vi "initalize 6221-2182-dc(SubVI).vi"(9 "字符串":string, 11 "簇":T13={"initialize"=enum."SR830", "6221"={"6221 Resource"="GPIB0::24::INSTR", "Delta status"=FALSE, "电流"=0.0}, "SR830+6221"={"source"=0, "阻抗"=0.0, "量程入 4"=0, "量程入 3"=0, "量程入 2"=0, "量程入 1"=0, "SR830 2"=FALSE, "SR830 3"=FALSE, "SR830 4"=FALSE, "SR830 1"=FALSE, "VISA 1"="", "VISA 2"="", "VISA 3"="", "VISA 4"="", "Reserve 1"=0, "Reserve 2"=-1, "Reserve 3"=-1, "Reserve 4"=-1, "量程"=enum."量程每次测量会判定"}, "2400"={"2400"=FALSE, "VISA"=""}, "ch"={"ch"=[], "current"=[], "change?"=[], "holding current\nwhen change ch?"=FALSE}, "Instrument"={"335 Resource"="GPIB0::24::INSTR", "Input (0:A)"=0, "Instrument Type"=enum."SVSM", "quantum design"=refnum, "Heater Output (1:1)"=1, "semaphore"=refnum, "TCP master instance"=refnum, "335 Status"=refnum, "M24C Resource"="GPIB0::24::INSTR", "4G supply"="GPIB0::24::INSTR", "Temp Status 24C"=refnum, "Temp"=refnum, "9T信号"=refnum, "limit"={"Field limit"=0.0, "Field rate limit"=0.0, "Temp limit"=0.0, "Temp low limit"=0.0, "Temp rate limit "=0.0}, "4g supply status"=refnum, "vi路径"=""}, "Aborting"=refnum, "数据文件"=refnum, "warning"=refnum, "2614B"={"2614B chA"=FALSE, "2614B chB"=FALSE, "VISA"=""}} {"Instrument"."Input (0:A)" items=["A", "B"]; "Instrument"."Heater Output (1:1)" items=["1"=1, "2"=2]; "SR830+6221"."Reserve 4" items=["Auto Reserve"=-1, "High Reserve"=0, "Normal"=1, "Low Noise"=2]; "SR830+6221"."Reserve 3" items=["Auto Reserve"=-1, "High Reserve"=0, "Normal"=1, "Low Noise"=2]; "SR830+6221"."Reserve 2" items=["Auto Reserve"=-1, "High Reserve"=0, "Normal"=1, "Low Noise"=2]; "SR830+6221"."Reserve 1" items=["量程每次测量会判定", "量程不变为设定值"]; "SR830+6221"."source" items=["SR830 1", "SR830 2", "SR830 3", "SR830 4"]}) -> (3 "输出簇":T13={"initialize"=enum."SR830", "6221"={"6221 Resource"="GPIB0::24::INSTR", "Delta status"=FALSE, "电流"=0.0}, "SR830+6221"={"source"=0, "阻抗"=0.0, "量程入 4"=0, "量程入 3"=0, "量程入 2"=0, "量程入 1"=0, "SR830 2"=FALSE, "SR830 3"=FALSE, "SR830 4"=FALSE, "SR830 1"=FALSE, "VISA 1"="", "VISA 2"="", "VISA 3"="", "VISA 4"="", "Reserve 1"=0, "Reserve 2"=-1, "Reserve 3"=-1, "Reserve 4"=-1, "量程"=enum."量程每次测量会判定"}, "2400"={"2400"=FALSE, "VISA"=""}, "ch"={"ch"=[], "current"=[], "change?"=[], "holding current\nwhen change ch?"=FALSE}, "Instrument"={"335 Resource"="GPIB0::24::INSTR", "Input (0:A)"=0, "Instrument Type"=enum."SVSM", "quantum design"=refnum, "Heater Output (1:1)"=1, "semaphore"=refnum, "TCP master instance"=refnum, "335 Status"=refnum, "M24C Resource"="GPIB0::24::INSTR", "4G supply"="GPIB0::24::INSTR", "Temp Status 24C"=refnum, "Temp"=refnum, "9T信号"=refnum, "limit"={"Field limit"=0.0, "Field rate limit"=0.0, "Temp limit"=0.0, "Temp low limit"=0.0, "Temp rate limit "=0.0}, "4g supply status"=refnum, "vi路径"=""}, "Aborting"=refnum, "数据文件"=refnum, "warning"=refnum, "2614B"={"2614B chA"=FALSE, "2614B chB"=FALSE, "VISA"=""}} {"Instrument"."Input (0:A)" items=["A", "B"]; "Instrument"."Heater Output (1:1)" items=["1"=1, "2"=2]; "SR830+6221"."Reserve 4" items=["Auto Reserve"=-1, "High Reserve"=0, "Normal"=1, "Low Noise"=2]; "SR830+6221"."Reserve 3" items=["Auto Reserve"=-1, "High Reserve"=0, "Normal"=1, "Low Noise"=2]; "SR830+6221"."Reserve 2" items=["Auto Reserve"=-1, "High Reserve"=0, "Normal"=1, "Low Noise"=2]; "SR830+6221"."Reserve 1" items=["量程每次测量会判定", "量程不变为设定值"]; "SR830+6221"."source" items=["SR830 1", "SR830 2", "SR830 3", "SR830 4"]})   [LabVIEW 2019, in "initialize.lvlib"]
uses:
  initialize.lvlib
  config.ctl
  <vilib>/NI/Modbus Library/API/Master/Modbus Master.lvclass
  initialize.ctl
  Instrument.ctl
  Instrument Type.ctl
  lib/QDInstrument.dll
  335 state.ctl
  limit.ctl
  9T mag field stauts.ctl
  warning.ctl
  lib/Keithley 622x/Configure/Source/Typedefs/KE622x -- Current Range.ctl
  lib/Keithley 622x/Configure/Source/Typedefs/KE622x -- Current Ranges.ctl
  lib/Keithley 622x/Typedefs/KE622x -- On Off Control.ctl
  lib/Keithley 622x/Configure/Output/Typedefs/KE6221 -- Output Response.ctl
  lib/Keithley 622x/Configure/Source/Typedefs/KE622x -- Current Level.ctl
  lib/Keithley 622x/Configure/Source/Typedefs/KE622x -- Voltage Limit.ctl
  lib/Keithley 622x/Configure/2182 -A/Low Level/Typedefs/KE2182 -- Voltage Ranges.ctl
  lib/Keithley 622x/Configure/2182 -A/Low Level/Typedefs/KE2182 -- Filter Type.ctl
  lib/Keithley 622x/Configure/2182 -A/Low Level/Typedefs/KE2182 -- Filter Count.ctl
  lib/Keithley 622x/Configure/2182 -A/Low Level/Typedefs/KE2182 -- Filter Window.ctl
  lib/Keithley 622x/Configure/2182 -A/Low Level/Typedefs/KE2182 -- NPLCs.ctl
  lib/Keithley 622x/Utility/Typedefs/KE622x -- Instrument Type.ctl
  lib/Keithley 622x/Keithley 622x.lvlib
panel:
  in  "2812 -A Params In":T6={"Auto Range?"=FALSE, "Man / Selected\nRange"=enum."10mV", "Enable Digital\nFilter?"=FALSE, "Filter Type"=enum."Moving", "Filter Count"=10, "Filter\nWindow (%)"=0.01, "Enable Analog\nFilter?"=FALSE, "NPLCs"=5} {"Filter\nWindow (%)" min=0.0 max=10.0 step=0.01 format="%.2f"; "Filter Count" min=1 max=100; "NPLCs" min=1 max=10}
  in  "Turn Off Output If Voltage Limit?":bool=TRUE
  out "error out":errorcluster
  out "Voltage Limit?":bool
  out "Interlock Tripped?":bool
  in  "Voltage Limit (V)":T7=10.0 min=0.1 max=105.0 step=0.01 format="%.2p"
  in  "Current Level (A)":T8=0.001 min=-0.105 max=0.105 format="%.4p"
  in  "Output Response":T9=enum."Slow"
  in  "Analog Filter State":T10
  in  "Current Range In":T11={"Auto Range?"=TRUE, "Man / Selected\nRange"=enum."2nA"}
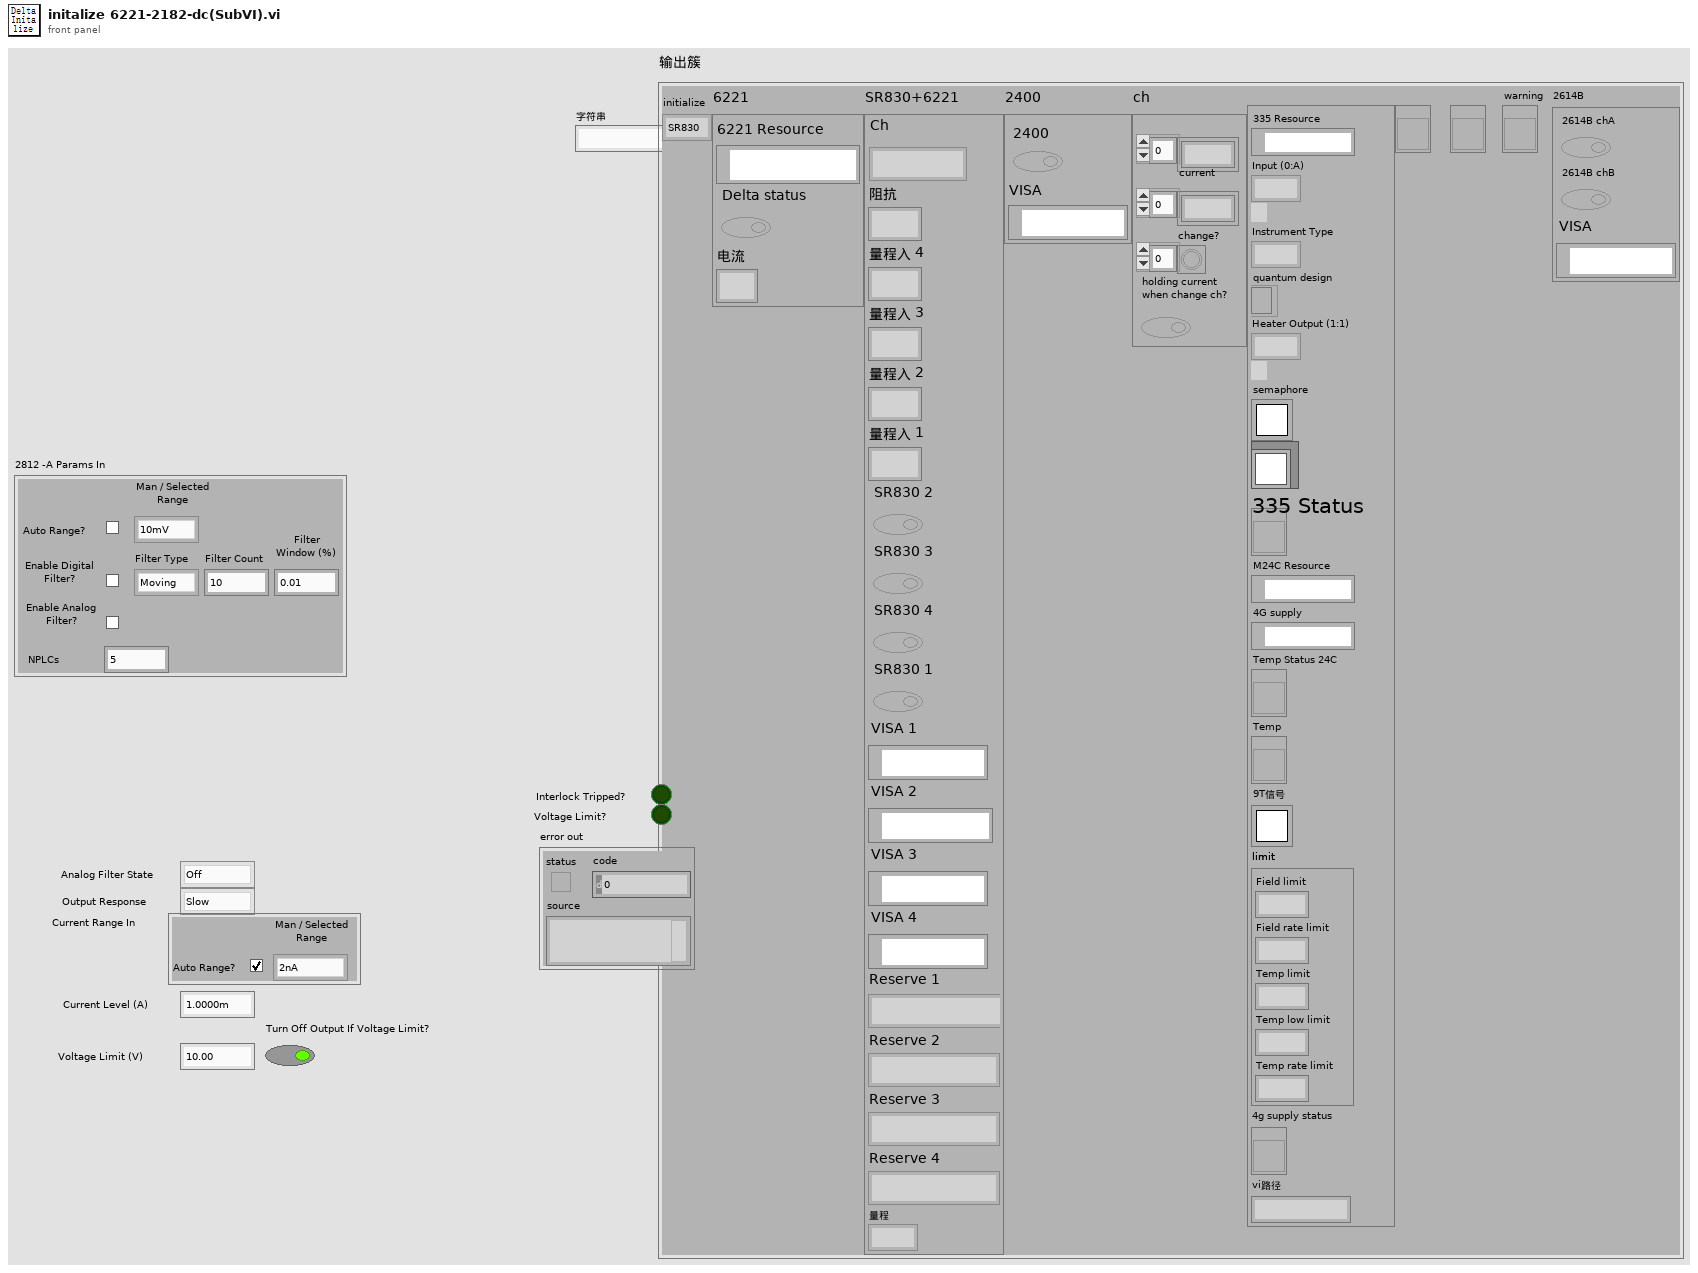
[diagram p1: front panel]
types:
  T1 = typedef "Keithley 622x.lvlib/KE2182 -- Voltage Ranges.ctl" = enum16{"10mV", "100mV", "1V", "10V", "100V"}
  T2 = typedef "Keithley 622x.lvlib/KE2182 -- Filter Type.ctl" = enum16{"Moving", "Repeat"}
  T3 = typedef "Keithley 622x.lvlib/KE2182 -- Filter Count.ctl" = u32
  T4 = typedef "Keithley 622x.lvlib/KE2182 -- Filter Window.ctl" = dbl
  T5 = typedef "Keithley 622x.lvlib/KE2182 -- NPLCs.ctl" = u32
  T6 = cluster{"Auto Range?":bool, "Man / Selected\nRange":T1, "Enable Digital\nFilter?":bool, "Filter Type":T2, "Filter Count":T3, "Filter\nWindow (%)":T4, "Enable Analog\nFilter?":bool, "NPLCs":T5}
  T7 = typedef "Keithley 622x.lvlib/KE622x -- Voltage Limit.ctl" = dbl
  T8 = typedef "Keithley 622x.lvlib/KE622x -- Current Level.ctl" = dbl
  T9 = typedef "Keithley 622x.lvlib/KE6221 -- Output Response.ctl" = enum16{"Fast", "Slow"}
  T10 = typedef "Keithley 622x.lvlib/KE622x -- On Off Control.ctl" = enum16{"Off", "On"}
  T11 = typedef "Keithley 622x.lvlib/KE622x -- Current Range.ctl" = cluster{"Auto Range?":bool, "Man / Selected\nRange":T12}
  T12 = typedef "Keithley 622x.lvlib/KE622x -- Current Ranges.ctl" = enum16{"2nA", "20nA", "200nA", "2uA", "20uA", "200uA", "2mA", "20mA", "100mA"}
  T13 = typedef "config.ctl" = cluster{"initialize":T14, "6221":cluster{"6221 Resource":refnum<visa-resource-name>, "Delta status":bool, "电流":dbl}, "SR830+6221":cluster{"source":u16, "阻抗":dbl, "量程入 4":i32, "量程入 3":i32, "量程入 2":i32, "量程入 1":i32, "SR830 2":bool, "SR830 3":bool, "SR830 4":bool, "SR830 1":bool, "VISA 1":refnum<visa-resource-name>, "VISA 2":refnum<visa-resource-name>, "VISA 3":refnum<visa-resource-name>, "VISA 4":refnum<visa-resource-name>, "Reserve 1":i16, "Reserve 2":i16, "Reserve 3":i16, "Reserve 4":i16, "量程":enum16{"量程每次测量会判定", "量程不变为设定值"}}, "2400":cluster{"2400":bool, "VISA":refnum<visa-resource-name>}, "ch":cluster{"ch":i32[], "current":dbl[], "change?":bool[], "holding current\nwhen change ch?":bool}, "Instrument":T15, "Aborting":refnum<vi>, "数据文件":refnum<vi>, "warning":refnum<vi>, "2614B":cluster{"2614B chA":bool, "2614B chB":bool, "VISA":refnum<visa-resource-name>}}
  T14 = typedef "initialize.ctl" = enum16{"SR830", "keithley6221-SR830", "Delta", "Delta-tunnelling", "keithley6221-2182-DC"}
  T15 = typedef "Instrument.ctl" = cluster{"335 Resource":refnum<visa-resource-name>, "Input (0:A)":u16, "Instrument Type":T16, "quantum design":refnum<k24>, "Heater Output (1:1)":u16, "semaphore":T17, "TCP master instance":refnum<class "Modbus Master.lvclass">, "335 Status":refnum<vi>, "M24C Resource":refnum<visa-resource-name>, "4G supply":refnum<visa-resource-name>, "Temp Status 24C":refnum<vi>, "Temp":refnum<vi>, "9T信号":T17, "limit":T18, "4g supply status":refnum<vi>, "vi路径":string}
  T16 = typedef "Instrument Type.ctl" = enum16{"PPMS", "VersaLab", "DynaCool", "SVSM", "PPMS-Rotate", "Lakeshore335", "9T mag"}
  T17 = typedef "Semaphore RefNum" = refnum<k1>
  T18 = typedef "limit.ctl" = cluster{"Field limit":dbl, "Field rate limit":dbl, "Temp limit":dbl, "Temp low limit":dbl, "Temp rate limit ":dbl}
  T19 = typedef "Keithley 622x.lvlib/KE622x -- Instrument Type.ctl" = enum16{"KE6220", "KE6221"}
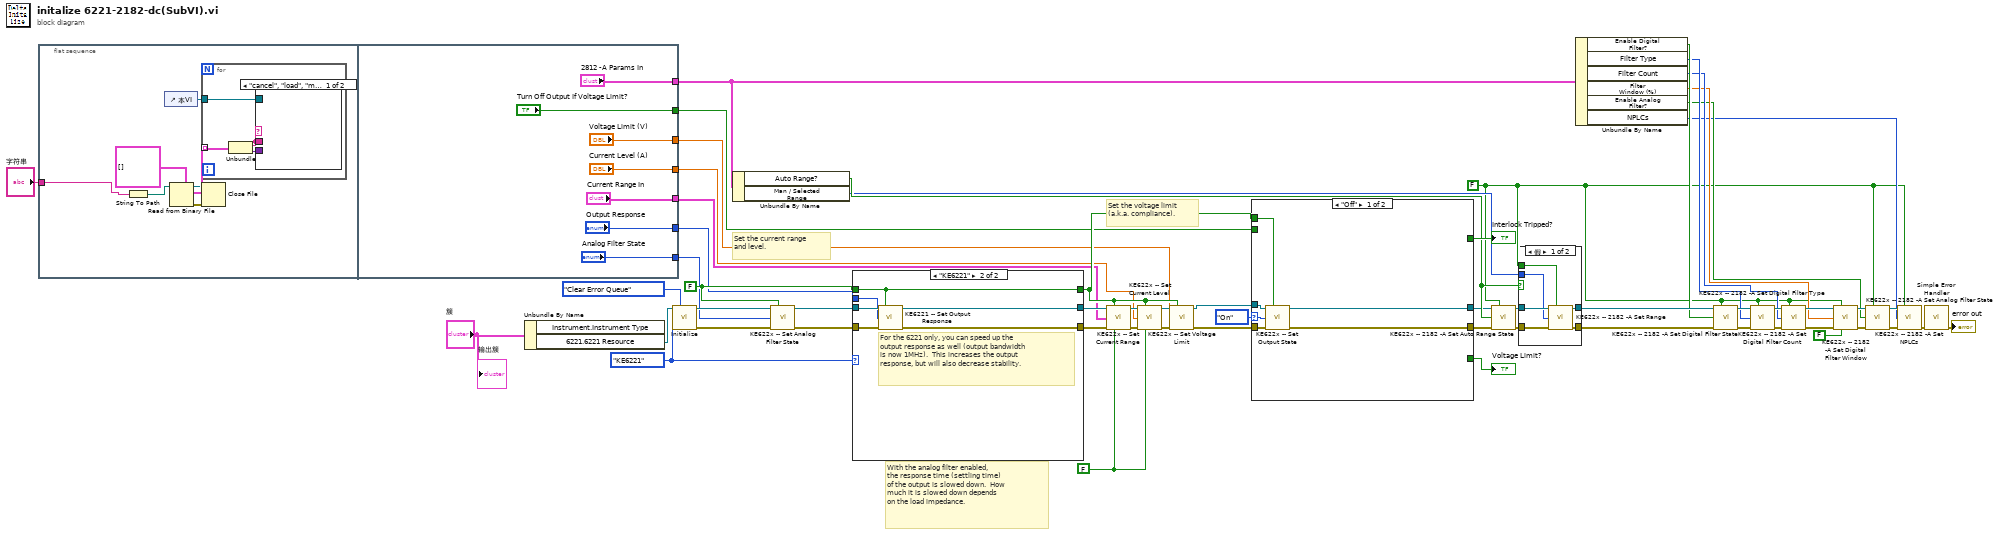
[diagram p0: block diagram]
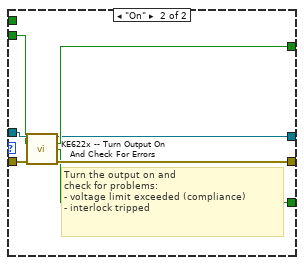
[diagram p3: hidden frame]
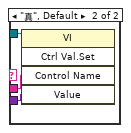
[diagram p5: hidden frame]
diagram:
  w7 = FALSE ("Check For SCPI Errors? (T)")
  w53 = KE622x_--_Instrument_Type."KE6221" ("Instrument Type")
  w51 = FALSE ("Check For SCPI Errors? (T)")
  w46 = FALSE ("Read Back Set Values? (T)")
  # "Set the voltage limit\n(a.k.a. compliance)."
  # "Set the current range\nand level."
  # "With the analog filter enabled,\nthe response time (settling time)\nof the output is slowed down.  How\nmuch it is slowed down depends\non the load impedance."
  n1 = flat-sequence {
    tunnel: "字符串" -> [w59]
    tunnel: ["Current Range In"] -> w36
    tunnel: ["Analog Filter State"] -> w35
    tunnel: ["Output Response"] -> w34
    tunnel: ["Voltage Limit (V)"] -> w33
    tunnel: ["Current Level (A)"] -> w32
    tunnel: ["Turn Off Output If Voltage Limit?"] -> w31
    tunnel: ["2812 -A Params In"] -> w6
    frame #0 {
      n2 = String To Path(string=w59) -> (path=w64:path)
      n3 = control-ref of="本VI"() -> (w65:refnum<vi>)
      n4 = Read from Binary File(5:cluster{"Name":string, "Variant Data":variant}[] [] ("控件值:获取全部"), 11:w64) -> (0:w60:errorcluster, 2:w62:cluster{"Name":string, "Variant Data":variant}[], 3:w61:refnum<file>)  [unwired: 4 in, 1 out]
      n5 = for {
        tunnel: w62 -> [w69] mode=indexing
        tunnel: w65 -> [w68]
        n6 = Unbundle(w69) -> ("Name"=w66:string, "Variant Data"=w67:variant)
        n7 = case shown="\"cancel\", \"load\", \"model\", \"ok\"" w66 {
          tunnel: w68 -> [_ w72]
          tunnel: w66 -> [_ w71]
          tunnel: w67 -> [_ w70]
          frame "cancel", "load", "model", "ok" {
          }
          frame "真", Default {
            n8 = invoke class="VI" method="Ctrl Val.Set"(reference=w72, "Control Name"=w71, "Value"=w70) -> ()  [unwired: 2 in, 5 out]
          }
        }
      }
      n9 = Close File(refnum=w61, error in=w60) -> ()  [unwired: 2 out]
    }
    frame #1 {
    }
  }
  n10 = Unbundle By Name("簇") -> ("6221.6221 Resource"=w1:refnum<visa-resource-name>)  [unwired: 1 out]
  n11 = call "Initialize.vi"("VISA resource name"=w1, "Error Queue Option"=enum16{"Clear Error Queue", "Error Query"}."Clear Error Queue", "Instrument Type"=w53) -> ("VISA resource name out"=w56:refnum<visa-resource-name>, "error out"=w55:errorcluster)  [unwired: 11 in]
  n12 = Unbundle By Name(w6) -> ("Auto Range?"=w16:bool, "Man / Selected\nRange"=w15:T1)
  n13 = call "KE622x -- Set Analog Filter State.vi"("Resource In"=w56, "Check For SCPI Errors? (T)"=w51, "Analog Filter State"=w35, "error in (no error)"=w55) -> ("Resource Out (dupl)"=w54:refnum<visa-resource-name>, "error out"=w52:errorcluster)  [unwired: 10 in]
  n14 = case shown="\"KE6221\"" w53 {
    tunnel: w54 -> [w81 w88]
    tunnel: w52 -> [w80 w87]
    tunnel: [w81 w86] -> w49
    tunnel: w51 -> [w82 w85]
    tunnel: [w82 w85] -> w39
    tunnel: [w80 w84] -> w50
    tunnel: w34 -> [_ w83]
    frame "KE6220" {
    }
    frame "KE6221" {
      # "For the 6221 only, you can speed up the\noutput response as well (output bandwidth\nis now 1MHz).  This increases the output\nresponse, but will also decrease stability."
      n15 = call "KE6221 -- Set Output Response.vi"("Resource In"=w88, "Check For SCPI Errors? (T)"=w85, "KE6221 Output Response"=w83, "error in (no error)"=w87) -> ("Resource Out (dupl)"=w86:refnum<visa-resource-name>, "error out"=w84:errorcluster)  [unwired: 10 in]
    }
  }
  n16 = call "KE622x -- Set Current Range.vi"("Resource In"=w49, "Check For SCPI Errors? (T)"=w39, "Current Range In"=w36, "error in (no error)"=w50, "Read Back Set Values? (T)"=w46) -> ("Resource Out (dupl)"=w48:refnum<visa-resource-name>, "error out"=w47:errorcluster)  [unwired: 8 in, 1 out]
  n17 = call "KE622x -- Set Current Level.vi"("Resource In"=w48, "Check For SCPI Errors? (T)"=w39, "Current Level (A) In"=w32, "error in (no error)"=w47, "Read Back Set Value? (T)"=w46) -> ("Resource Out (dupl)"=w45:refnum<visa-resource-name>, "error out"=w44:errorcluster)  [unwired: 8 in, 1 out]
  n18 = call "KE622x -- Set Voltage Limit.vi"("Resource In"=w45, "Check For SCPI Errors? (T)"=w39, "Voltage Limit (V)"=w33, "error in (no error)"=w44) -> ("Resource Out (dupl)"=w43:refnum<visa-resource-name>, "error out"=w42:errorcluster)  [unwired: 10 in]
  n19 = case shown="\"Off\"" KE622x_--_On_Off_Control."On" ("Output State") {
    selector: KE622x_--_On_Off_Control."On" ("Output State") -> [w92 _]
    tunnel: w43 -> [w94 w101]
    tunnel: w42 -> [w93 w100]
    tunnel: [w90 w99] -> w4
    tunnel: w39 -> [w91 _]
    tunnel: [_ w98] -> w38
    tunnel: [_ w97] -> w37
    tunnel: w31 -> [_ w96]
    tunnel: [w89 w95] -> w5
    frame "Off" {
      n20 = call "KE622x -- Set Output State.vi"("Resource In"=w94, "Check For SCPI Errors? (T)"=w91, "Output State"=w92, "error in (no error)"=w93) -> ("Resource Out (dupl)"=w89:refnum<visa-resource-name>, "error out"=w90:errorcluster)  [unwired: 10 in]
    }
    frame "On" {
      # "Turn the output on and\ncheck for problems:\n- voltage limit exceeded (compliance)\n- interlock tripped"
      n21 = call "KE622x -- Turn Output On And Check For Errors.vi"("Resource In"=w101, "Turn Off Output If Compliance?"=w96, "error in (no error)"=w100) -> ("Resource Out (dupl)"=w95:refnum<visa-resource-name>, "Interlock Tripped?"=w98:bool, "Compliance?"=w97:bool, "error out"=w99:errorcluster)  [unwired: 9 in]
    }
  }
  "Interlock Tripped?" <- w38
  "Voltage Limit?" <- w37
  n22 = call "KE622x -- 2182 -A Set Auto Range State.vi"("622x Resource In"=w5, "Check For SCPI Errors? (T)"=w7, "Enable Auto Range?"=w16, "error in (no error)"=w4) -> ("622x Resource Out (dupl)"=w30:refnum<visa-resource-name>, "error out"=w29:errorcluster)  [unwired: 10 in]
  n23 = case shown="假" w16 {
    tunnel: w30 -> [w107 w109]
    tunnel: w29 -> [w106 w108]
    tunnel: [w105 w109] -> w28
    tunnel: [w104 w108] -> w27
    tunnel: w15 -> [w102 _]
    tunnel: w7 -> [w103 _]
    frame False {
      n24 = call "KE622x -- 2182 -A Set Range.vi"("622x Resource In"=w107, "Check For SCPI Errors? (T)"=w103, "2182/2182A Range"=w102, "error in (no error)"=w106) -> ("622x Resource Out (dupl)"=w105:refnum<visa-resource-name>, "error out"=w104:errorcluster)  [unwired: 10 in]
    }
    frame True {
    }
  }
  n25 = Unbundle By Name(w6) -> ("Enable Digital\nFilter?"=w14:bool, "Filter Type"=w13:T2, "Filter Count"=w12:T3, "Filter\nWindow (%)"=w11:T4, "Enable Analog\nFilter?"=w10:bool, "NPLCs"=w9:T5)
  n26 = call "KE622x -- 2182 -A Set Digital Filter State.vi"("622x Resource In"=w28, "Check For SCPI Errors? (T)"=w7, "Enable Digital Filter?"=w14, "error in (no error)"=w27) -> ("622x Resource Out (dupl)"=w26:refnum<visa-resource-name>, "error out"=w25:errorcluster)  [unwired: 10 in]
  n27 = call "KE622x -- 2182 -A Set Digital Filter Type.vi"("622x Resource In"=w26, "Check For SCPI Errors? (T)"=w7, "Filter Type"=w13, "error in (no error)"=w25) -> ("622x Resource Out (dupl)"=w24:refnum<visa-resource-name>, "error out"=w23:errorcluster)  [unwired: 10 in]
  n28 = call "KE622x -- 2182 -A Set Digital Filter Count.vi"("622x Resource In"=w24, "Check For SCPI Errors? (T)"=w7, "Filter Count"=w12, "error in (no error)"=w23) -> ("622x Resource Out (dupl)"=w19:refnum<visa-resource-name>, "error out"=w22:errorcluster)  [unwired: 10 in]
  n29 = call "KE622x -- 2182 -A Set Digital Filter Window.vi"("622x Resource In"=w19, "Check For SCPI Errors? (T)"=w7, "Filter Window In (%)"=w11, "error in (no error)"=w22, "Read Back Set Value? (T)"=FALSE) -> ("622x Resource Out (dupl)"=w18:refnum<visa-resource-name>, "error out"=w21:errorcluster)  [unwired: 9 in]
  n30 = call "KE622x -- 2182 -A Set Analog Filter State.vi"("622x Resource In"=w18, "Check For SCPI Errors? (T)"=w7, "Enable Analog Filter?"=w10, "error in (no error)"=w21) -> ("622x Resource Out (dupl)"=w17:refnum<visa-resource-name>, "error out"=w20:errorcluster)  [unwired: 10 in]
  n31 = call "KE622x -- 2182 -A Set NPLCs.vi"("622x Resource In"=w17, "Check For SCPI Errors? (T)"=w7, "2182 -A NPLCs"=w9, "error in (no error)"=w20) -> ("error out"=w3:errorcluster)  [unwired: 10 in, 1 out]
  n32 = call <vilib>:"Simple Error Handler.vi"("error in (no error)"=w3) -> ("error out"=→"error out":errorcluster)  [unwired: 4 in, 4 out]
  "输出簇" <- "簇"
